vi "Override and Call.vi"(8 "error in (no error)":errorcluster, 11 "Child in":refnum<class "Child.lvclass">) -> (0 "error out":errorcluster, 3 "Child out":refnum<class "Child.lvclass">)   [LabVIEW 2021, in "Child.lvclass"]
uses:
  Child.lvclass
  Child.lvclass/Child.ctl
  Override and Call Interface/Override and Call Interface.lvclass
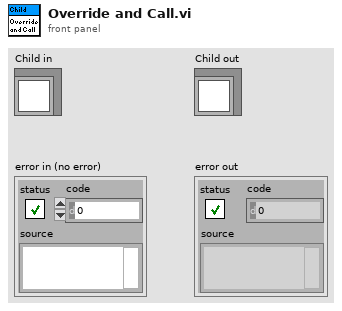
[diagram p1: front panel]
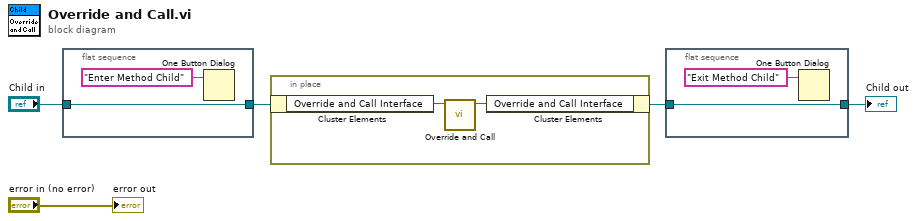
[diagram p0: block diagram]
diagram:
  n1 = flat-sequence {
    tunnel: [w6] -> w3
    tunnel: "Child in" -> [w6]
    frame #0 {
      n2 = One Button Dialog(message="Enter Method Child") -> ()  [unwired: 1 in, 1 out]
    }
  }
  n3 = in-place {
    n4 = in-place-cluster #1(w3) -> ("Override and Call Interface"=w9:refnum<class "Override and Call Interface.lvclass">)
    n5 = call-dynamic "Override and Call.vi"("Override and Call Interface in"=w9) -> ("Override and Call Interface out"=w8:refnum<class "Override and Call Interface.lvclass">)  [unwired: 9 in, 1 out]
    n6 = in-place-cluster #1("Override and Call Interface"=w8) -> (w2:refnum<class "Child.lvclass">)
  }
  n7 = flat-sequence {
    tunnel: [w10] -> w1
    tunnel: w2 -> [w10]
    frame #0 {
      n8 = One Button Dialog(message="Exit Method Child") -> ()  [unwired: 1 in, 1 out]
    }
  }
  "error out" <- "error in (no error)"
  "Child out" <- w1
